vi "Create New File.vi"(8 "Filename Suffix (_data.csv)":string="_data.csv", 9 "Time Format String\n(%y_%m_%d__%H_%M_%S%4u)":string="%y_%m_%d__%H_%M_%S%4u", 10 "Output Directory":path=path "C:/Users/Josh/Desktop/code/CVB/Config/generated_data", 11 "Create New File":bool=TRUE) -> (3 "Output Filename":path)   [LabVIEW 2021]
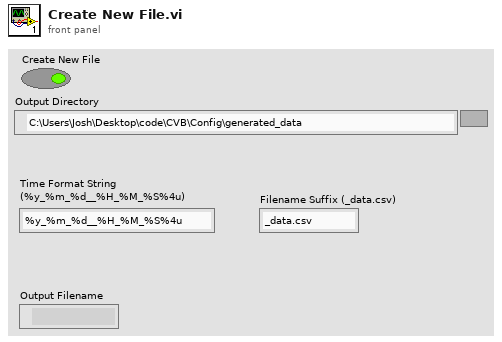
[diagram p1: front panel]
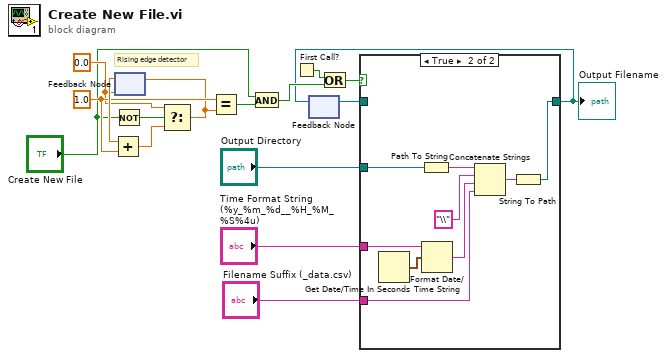
[diagram p0: block diagram]
diagram:
  w12 = 0.0
  w15 = 1.0 ("y")
  # "Rising edge detector"
  n1 = Not(x="Create New File") -> (.not. x?=w10:bool)
  n2 = feedback #1(w12) -> (w16:dbl)
  n3 = Add(x=w16, y=w15) -> (x+y=w11:dbl)
  n4 = Select(t=w12, s=w10, f=w11) -> (s? t:f=w13:dbl)
  n5 = feedback-in #1(w13) -> ()
  n6 = Equal?(x=w15, y=w13) -> (x = y?=w14:bool)
  n7 = And(x="Create New File", y=w14) -> (x .and. y?=w7:bool)
  n8 = First Call?() -> (First Call?: T/F=w6:bool)
  n9 = feedback #2() -> (w5:path)  [unwired: 1 in]
  n10 = Or(x=w6, y=w7) -> (x .or. y?=w8:bool)
  n11 = case shown="True" w8 {
    tunnel: [w17 w26] -> w4
    tunnel: w5 -> [w17 _]
    tunnel: "Output Directory" -> [_ w20]
    tunnel: "Time Format String\n(%y_%m_%d__%H_%M_%S%4u)" -> [_ w19]
    tunnel: "Filename Suffix (_data.csv)" -> [_ w18]
    frame False {
    }
    frame True {
      n12 = Get Date/Time In Seconds() -> (seconds since 1Jan1904=w21:timestamp)
      n13 = Path To String(path=w20) -> (string=w24:string)
      n14 = Format Date/Time String(time format string (%c)=w19, seconds (now)=w21) -> (date/time string=w23:string)  [unwired: 1 in]
      n15 = Concatenate Strings(w24, "\\" ("string"), w23, w18) -> (w22:string)
      n16 = String To Path(string=w22) -> (path=w26:path)
    }
  }
  "Output Filename" <- w4
  n17 = feedback-in #2(w4) -> ()
